vi "read_1_byte_SubVI.vi"(10 "min time SCL Low (uSEC)":u32, 11 "min time SCL High (uSEC)":u32) -> (3 "Data bit array":bool[](array[boolean]))   [LabVIEW 2019]
panel:
  out "ACK":bool
  out "NMAK":bool
  in  "Last byte ?":bool
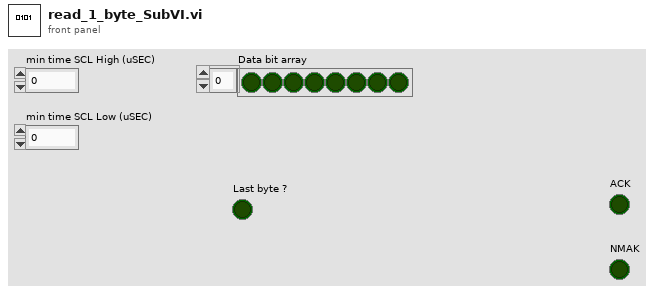
[diagram p1: front panel]
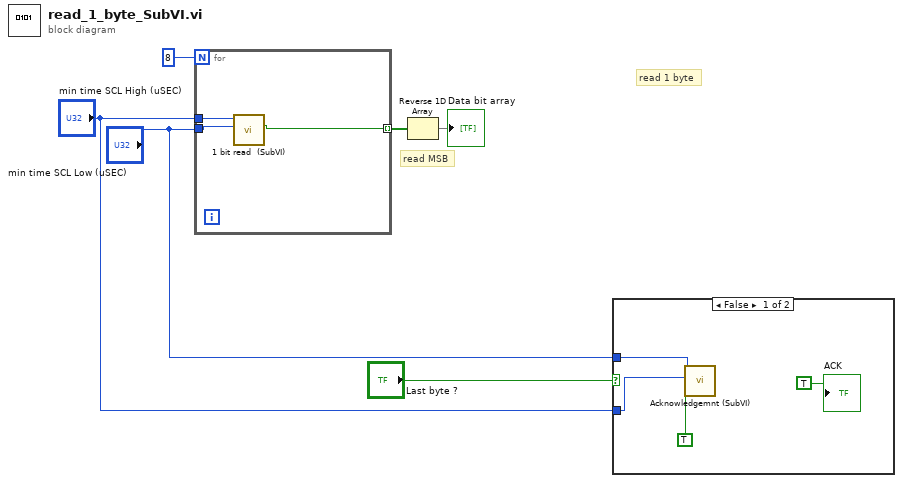
[diagram p0: block diagram]
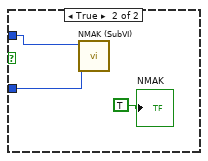
[diagram p2: hidden frame]
diagram:
  # "read 1 byte"
  # "read MSB"
  n1 = for {
    N: 8 -> [_]
    tunnel: "min time SCL High (uSEC)" -> [w9]
    tunnel: "min time SCL Low (uSEC)" -> [w8]
    tunnel: [w7] -> w5 mode=indexing
    n2 = call "1 bit read  (SubVI).vi"("min time SCL Low (uSEC)"=w8, "min time SCL High (uSEC)"=w9) -> ("Data bit"=w7:bool)  [unwired: 9 in]
  }
  n3 = Reverse 1D Array(array=w5) -> (reversed array=→"Data bit array":bool[])
  n4 = case shown="False" "Last byte ?" {
    tunnel: "min time SCL Low (uSEC)" -> [w12 w16]
    tunnel: "min time SCL High (uSEC)" -> [w11 w15]
    frame False {
      n5 = call "Acknowledgemnt (SubVI).vi"("Acknowledgement"=TRUE, "min time SCL High (uSEC)"=w11, "min time SCL Low (uSEC)"=w12) -> ()  [unwired: 9 in]
      "ACK" <- TRUE
    }
    frame True {
      n6 = call "NMAK (SubVI).vi"("min time SCL High (uSEC)"=w15, "min time SCL Low (uSEC)"=w16) -> ()  [unwired: 10 in]
      "NMAK" <- TRUE
    }
  }
